vi "Mutexed Publish Data.vi"(4 "Return Error Transport":refnum<class "ITransport.lvclass">, 6 "Publish Time (Use Current Time)":timestamp, 7 "PublicationPolicy":refnum<class "IPublicationPolicy.lvclass">, 8 "error in (no error)":errorcluster, 9 "Numeric Type":variant, 10 "Datum Name":string, 11 "IModel in":refnum<class "IModel.lvclass">) -> (0 "error out":errorcluster, 3 "IModel out":refnum<class "IModel.lvclass">)   [LabVIEW 2017, in "IModel.lvlib" / "IModel.lvclass"]
doc: "Publish a datum (value) to the mediator bus. Published data are observable by any actor with access to the mediated bus."
uses:
  IModel.lvclass
  C:/Git/mva-framework/Framework/IObserver/IObserver/IObserver.lvclass
  IMediator/IPublicationPolicy/IPublicationPolicy.lvclass
  IMediator/ITransport/ITransport.lvclass
  <vilib>/ActorFramework/Actor/Actor.lvclass/Actor.ctl
  <vilib>/ActorFramework/Message Enqueuer/Message Enqueuer.lvclass/Message Enqueuer.ctl
  IMediator/PublishRequest/PublishRequest.lvclass/PublishRequest.ctl
  IMediator/MutexedPublishRequest/MutexedPublishRequest.lvclass/MutexedPublishRequest.ctl
  IModel.lvclass/IModel.ctl
  AbstractMessages/PreAddressedMsg/PreAddressedMsg.lvclass/PreAddressedMsg.ctl
  IMediator/IMediator Messages/Publish Msg/Publish Msg.lvclass/Publish Msg.ctl
  IMediator/PublishRequest/Write Publish Request Data.vi
  <vilib>/ActorFramework/Message Enqueuer/Enqueue.vi
  AbstractMessages/PreAddressedMsg/Read Return Address.vi
  <vilib>/ActorFramework/Actor/Read Self Enqueuer.vi
  <vilib>/ActorFramework/Message Enqueuer/Init from Existing Queue.vi
  IObserver/IObserver/IObserver.lvclass
  C:/Program Files (x86)/National Instruments/LabVIEW 2017/vi.lib/ActorFramework/Actor/Actor.lvclass
  IMediator/MutexedPublishRequest/MutexedPublishRequest.lvclass
  C:/Git/mva-framework/Framework/IMediator/PublishRequest/PublishRequest.lvclass
  IMediator/IMediator Messages/Publish Msg/Publish Msg.lvclass
  C:/Git/mva-framework/Framework/AbstractMessages/PreAddressedMsg/PreAddressedMsg.lvclass
  C:/Program Files (x86)/National Instruments/LabVIEW 2017/vi.lib/ActorFramework/Message/Message.lvclass
  <vilib>/ActorFramework/Message Priority Queue/Priority Enqueue.vi
  <vilib>/ActorFramework/Message Enqueuer/Message Enqueuer.lvclass
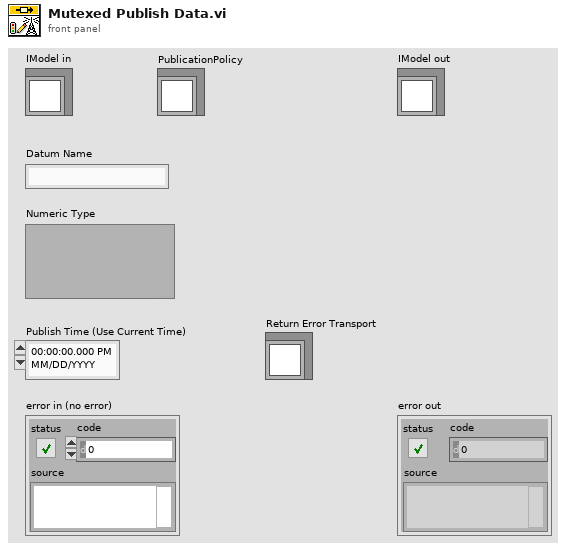
[diagram p1: front panel]
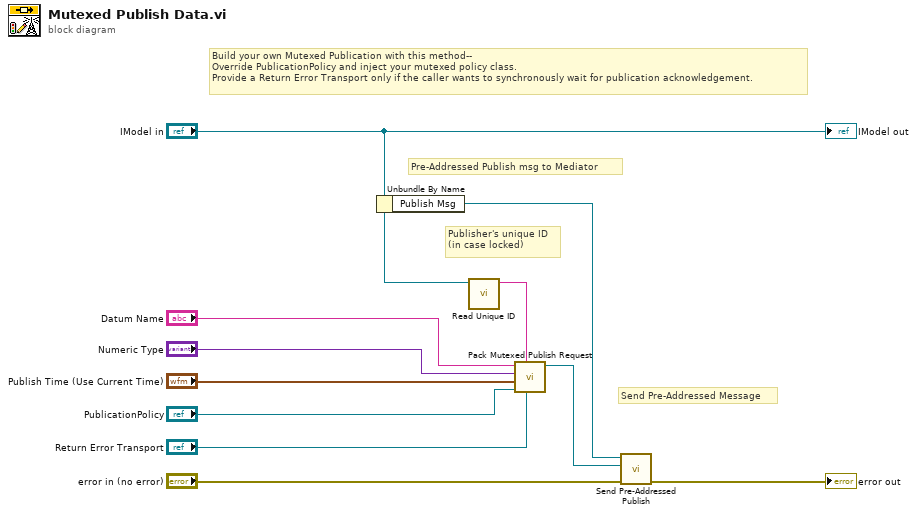
[diagram p0: block diagram]
diagram:
  # "Publisher's unique ID\n(in case locked)"
  # "Pre-Addressed Publish msg to Mediator"
  # "Send Pre-Addressed Message"
  # "Build your own Mutexed Publication with this method--\nOverride PublicationPolicy and inject your mutexed policy class.\nProvide a Return Error Transport only if the caller wants to synchronously wait for publication acknowledgement."
  n1 = Unbundle By Name("IModel in") -> ("Publish Msg"=w3:refnum<class "Publish Msg.lvclass">)
  n2 = call "Read Unique ID.vi"("IObserver In"="IModel in") -> ("Unique ID"=w1:string)  [unwired: 10 in]
  n3 = call "Pack Mutexed Publish Request.vi"("Return Error Transport"="Return Error Transport", "Publisher ID"=w1, "PublicationPolicy"="PublicationPolicy", "Publish Time (Use Current Time)"="Publish Time (Use Current Time)", "Datum Value or Type"="Numeric Type", "Datum Name"="Datum Name") -> ("MutexedPublishRequest Out"=w2:refnum<class "MutexedPublishRequest.lvclass">)  [unwired: 5 in]
  n4 = call "Send Pre-Addressed Publish.vi"("error in (no error)"="error in (no error)", "PublishRequest"=w2, "Publish Message"=w3) -> ("error out"=→"error out":errorcluster)  [unwired: 8 in]
  "IModel out" <- "IModel in"
